vi "WriteToFIFOPort3.vi"() -> ()   [LabVIEW 2011]
doc: "Elizabeth Mahon\nMore or less just a copy of its port1 counterpart, which worked in testing. Check there for further notes.\nThis one has not yet been tested.s"
uses:
  <vilib>/LabVIEW Targets/FPGA/cRIO/shared/nicrio_ModuleControls/nicrio_cRIO-9871_BaudRateEnum.ctl
  <vilib>/rvi/eio/common/nirviEmuTemplateMethod_errors.vi
  <vilib>/rvi/interface/RandomDataEmulation/nirviRandomDataFPGAFIFO.vi
  <vilib>/rvi/interface/RandomDataEmulation/niFpgaRandomDataHandleErrors.vi
  <vilib>/rvi/eio/common/nirviEmuTemplatePropertySet_noerrors.vi
  <vilib>/eio/EIOMethodNode/EIOMethodNode.xnode
  <vilib>/rvi/DataTransferAndStorage/Container/XNode/niFpgaContainer.xnode
  <vilib>/rvi/interface/RandomDataEmulation/nirviRandomDataFpgaReadWriteTemplate.vi
  <vilib>/eio/EIOPropertyNode/EIOPropertyNode.xnode
  <vilib>/rvi/eio/common/nirviEmuTemplatePropertyGet_errors.vi
  <vilib>/rvi/eio/common/nirviEmuTemplatePropertyGet_noerrors.vi
  <vilib>/rvi/eio/common/nirviEmuTemplatePropertySet_errors.vi
panel:
  in  "StopPort2":bool
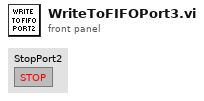
[diagram p1: front panel]
types:
  T1 = typedef "nicrio_cRIO-9871_BaudRateEnum.ctl" = enum16{"75 bps", "110 bps", "134 bps", "150 bps", "300 bps", "600 bps", "1200 bps", "1800 bps", "2400 bps", "4800 bps", "7200 bps", "9600 bps", "14.4 kbps", "19.2 kbps", "28.8 kbps", "38.4 kbps", "57.6 kbps", "115.2 kbps", "230.4 kbps", "460.8 kbps", "921.6 kbps"}
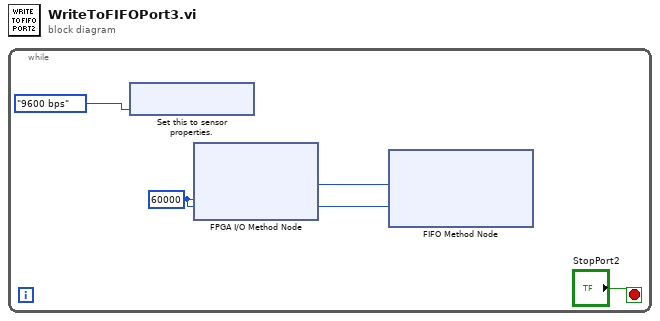
[diagram p0: block diagram]
diagram:
  n1 = while {
    stop <- "StopPort2" stop-if-true
    w2 = 60000 ("Timeout (ms)")
    n2 = xnode "Set this to sensor properties."("Baud Rate"=nicrio_cRIO-9871_BaudRateEnum."9600 bps") -> ()  [unwired: 1 in, 1 out]
    n3 = xnode "FPGA I/O Method Node"("Timeout (ms)"=w2) -> ("Data"=w3:u8)  [unwired: 1 in, 2 out]
    n4 = xnode ("FIFO Method Node")("Element"=w3, "Timeout"=w2) -> ()  [unwired: 1 in, 2 out]
  }
